vi "Initialize (SubVI).vi"(0 "path":path, 2 "error IN":errorcluster) -> (3 "pathConfigOUT":path, 4 "lengthUnits":string, 5 "massUnits":string, 6 "error out":errorcluster)   [LabVIEW 2015]
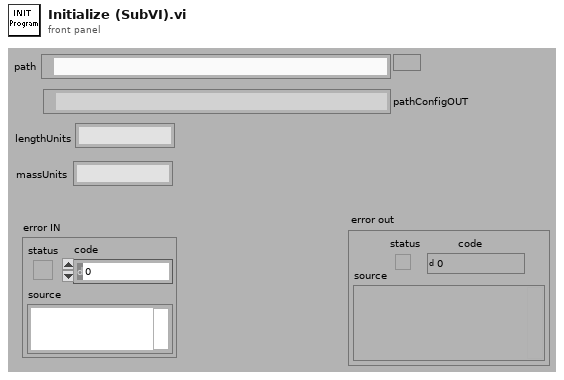
[diagram p1: front panel]
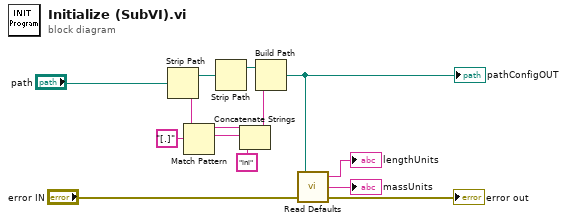
[diagram p0: block diagram]
diagram:
  n1 = Strip Path(path="path") -> (stripped path=w12:path, name=w10:string)
  n2 = Match Pattern(string=w10, regular expression="[.]") -> (before substring=w7:string, match substring=w6:string)  [unwired: 3 out]
  n3 = Strip Path(path=w12) -> (stripped path=w5:path)  [unwired: 1 out]
  n4 = Concatenate Strings(w7, w6, "ini" ("string")) -> (w9:string)
  n5 = Build Path(base path=w5, name or relative path=w9) -> (appended path=w4:path)
  "pathConfigOUT" <- w4
  n6 = call "Read Defaults.vi"("error in (no error)"="error IN", "appended path"=w4) -> ("error out"=→"error out":errorcluster, "massUnits"=→"massUnits":string, "lengthUnits"=→"lengthUnits":string)  [unwired: 1 out]
